vi "create socket.vi"(9 "lvsocket":u64, 10 "tls socket":u64, 11 "connection":refnum<k5>) -> (3 "lvlibretls connection out":refnum<class "lvlibretls connection.lvclass">)   [LabVIEW 2016, in "lvlibretls connection.lvclass"]
doc: "Generally for internal use only."
uses:
  lvlibretls connection.lvclass
  lvlibretls connection.lvclass/lvlibretls connection.ctl
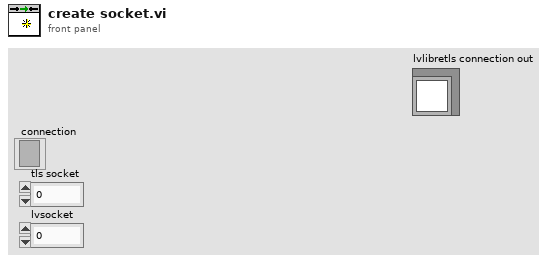
[diagram p1: front panel]
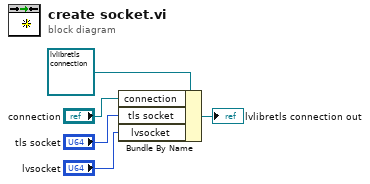
[diagram p0: block diagram]
diagram:
  n1 = Bundle By Name(cluster=refnum<class "lvlibretls connection.lvclass"> refnum ("lvlibretls connection in"), "connection"="connection", "tls socket"="tls socket", "lvsocket"="lvsocket") -> (→"lvlibretls connection out":refnum<class "lvlibretls connection.lvclass">)
